vi "Calculate Distance.vi"(9 "Mounting Angle":dbl, 10 "Height of LL":dbl=2.041667, 11 "Height of Target":dbl=8.1875) -> (1 "Raw Angle":dbl, 2 "Valid?":bool, 3 "Distance":dbl)   [LabVIEW 2019]
uses:
  <vilib>/Rock Robotics/Network Tables/NT Read Number.vi
panel:
  # "Height is in feet"
  # "Power Port total Height  = 120.1875 inches or 10.1875ft"
  # "Inner port height = 98.25 inches or 8.1875ft"
  # "LL height = 24.5 inches or 2.041667ft"
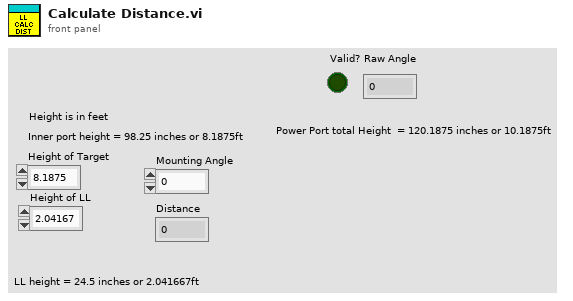
[diagram p1: front panel]
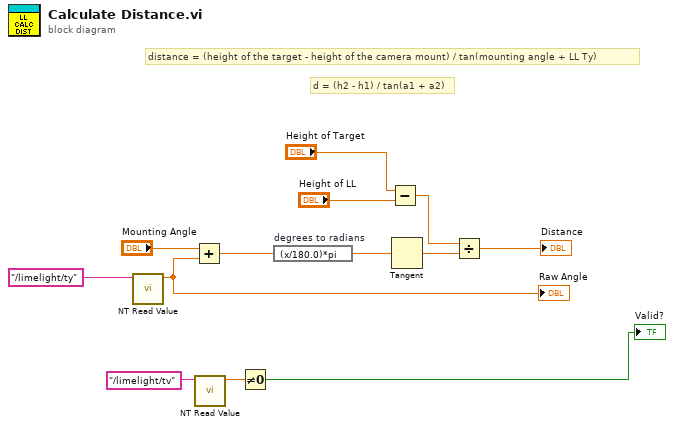
[diagram p0: block diagram]
diagram:
  # "d = (h2 - h1) / tan(a1 + a2)"
  # "distance = (height of the target - height of the camera mount) / tan(mounting angle + LL Ty)"
  n1 = call-poly <vilib>:"NT Read Value.vi"("Name"="/limelight/ty") -> ("Numeric"=w8:dbl)  [unwired: 9 in, 1 out]
  "Raw Angle" <- w8
  n2 = Add(x="Mounting Angle", y=w8) -> (x+y=w7:dbl)
  n3 = call-poly <vilib>:"NT Read Value.vi"("Name"="/limelight/tv") -> ("Numeric"=w2:dbl)  [unwired: 9 in, 1 out]
  n4 = Not Equal To 0?(x=w2) -> (x != 0?=→"Valid?":bool)
  n5 = expression code="(x/180.0)*pi" "degrees to radians"(w7) -> (w4:dbl)
  n6 = Subtract(x="Height of Target", y="Height of LL") -> (x-y=w11:dbl)
  n7 = Tangent(1:w4) -> (0:w5:dbl)
  n8 = Divide(x=w11, y=w5) -> (x/y=→"Distance":dbl)
